vi "例6-8.vi"() -> ()   [LabVIEW 2019]
uses:
  <vilib>/Analysis/2dsp.llb/1D Cross Correlation (DBL).vi
  <vilib>/Analysis/NI_AALBase.lvlib
  <vilib>/Analysis/NI_AALPro.lvlib
panel:
  in  "采样点数":dbl=100.0
  in  "采样频率":dbl=100.0
  in  "初始相位2":dbl
  in  "频率2":dbl=10.0
  in  "初始相位1":dbl
  in  "频率1":dbl=10.0
  out "相关后波形":dbl[](graph)
  out "信号波形":dbl[][](graph)
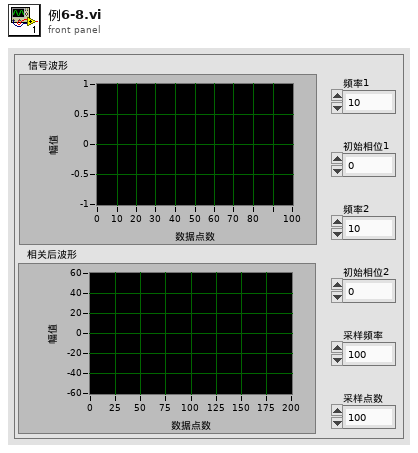
[diagram p1: front panel]
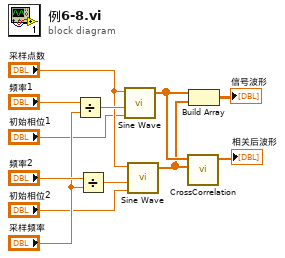
[diagram p0: block diagram]
diagram:
  n1 = Divide(x="频率1", y="采样频率") -> (x/y=w9:dbl)
  n2 = Divide(x="频率2", y="采样频率") -> (x/y=w8:dbl)
  n3 = call <vilib>:"Sine Wave.vi"("samples"="采样点数", "frequency"=w9, "phase in"="初始相位1") -> ("sine wave"=w3:dbl[])  [unwired: 2 in, 2 out]
  n4 = call <vilib>:"Sine Wave.vi"("samples"="采样点数", "frequency"=w8, "phase in"="初始相位2") -> ("sine wave"=w2:dbl[])  [unwired: 2 in, 2 out]
  n5 = call-poly <vilib>:"CrossCorrelation.vi"("Y"=w2, "X"=w3) -> ("Rxy"=→"相关后波形":dbl[])  [unwired: 8 in, 1 out]
  n6 = Build Array(w3, w2) -> (→"信号波形":dbl[][])
